vi "FL_SG_Filter_2.vi"(1 "N samples":i32, 2 "SG coefficients":dbl[](array[numeric]), 3 "Input sample":dbl format="%#_13g") -> (0 "Filtered sample":dbl)   [LabVIEW 2018]
doc: "This VI makes a Savitzky-Golay filtered of input data, length of the fitler is 31 sample, 3rd order polynom. First (and possibly last, depend on filter work mode) 15 values entered into filter will be filtered via simplified Klaman with K=0.3 instead."
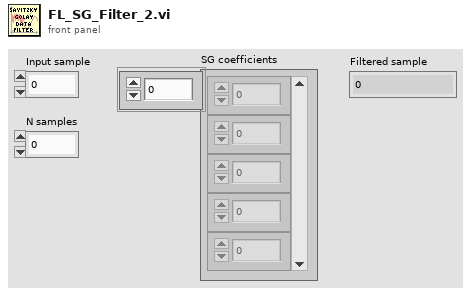
[diagram p1: front panel]
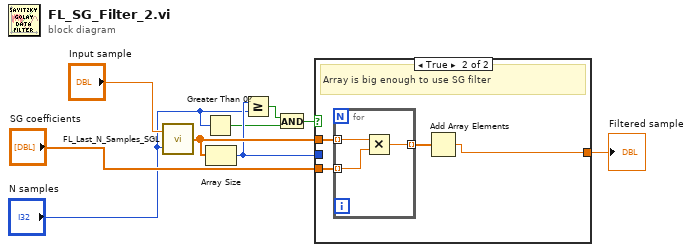
[diagram p0: block diagram]
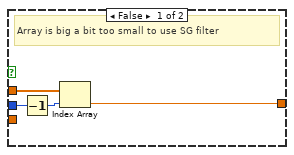
[diagram p2: hidden frame]
diagram:
  n1 = call "FL_Last_N_Samples_SGL.vi"("BufferLengthSamples"="N samples", "Input sample"="Input sample") -> ("Output Array"=w9:dbl[])
  n2 = Greater Than 0?(x="N samples") -> (x > 0?=w2:bool)
  n3 = Array Size(array=w9) -> (size(s)=w7:i32)
  n4 = Greater Or Equal?(x=w7, y="N samples") -> (x >= y?=w3:bool)
  n5 = And(x=w3, y=w2) -> (x .and. y?=w4:bool)
  n6 = case shown="True" w4 {
    tunnel: w9 -> [w13 w17]
    tunnel: "SG coefficients" -> [_ w16]
    tunnel: [w12 w14] -> w8
    tunnel: w7 -> [w11 _]
    frame False {
      # "Array is big a bit too small to use SG filter"
      n7 = Decrement(x=w11) -> (x-1=w10:i32)
      n8 = Index Array(array=w13, index=w10) -> (element=w12:dbl)
    }
    frame True {
      # "Array is big enough to use SG filter"
      n9 = for {
        tunnel: w17 -> [w20] mode=indexing
        tunnel: w16 -> [w18] mode=indexing
        tunnel: [w19] -> w15 mode=indexing
        n10 = Multiply(x=w20, y=w18) -> (x*y=w19:dbl)
      }
      n11 = Add Array Elements(numeric array=w15) -> (sum=w14:dbl)
    }
  }
  "Filtered sample" <- w8
